vi "Process.vi"(8 "error in (no error)":errorcluster, 10 "Start State in":refnum<class "Start State.lvclass">, 11 "Architecture.lvlib:Thread.lvclass":refnum<class "Thread.lvclass">) -> (0 "error out":errorcluster, 1 "Stop?":bool, 3 "Architecture.lvlib:Thread.lvclass 2":refnum<class "Thread.lvclass">)   [LabVIEW 2019, in "Car Wash Controller.lvlib" / "Start State.lvclass"]
uses:
  Start State.lvclass
  Message/Message.lvclass
  Thread/Thread.lvclass
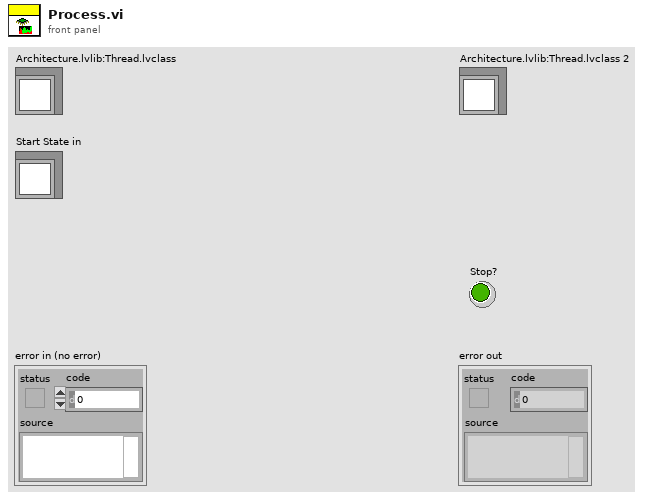
[diagram p1: front panel]
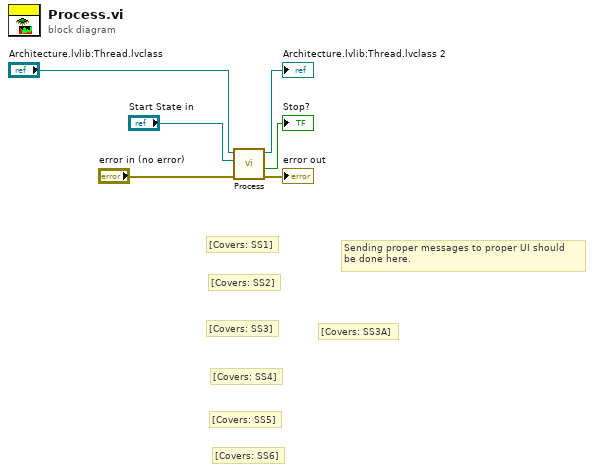
[diagram p0: block diagram]
diagram:
  # "[Covers: SS3A]"
  # "Sending proper messages to proper UI should\nbe done here."
  # "[Covers: SS6]"
  # "[Covers: SS5]"
  # "[Covers: SS4]"
  # "[Covers: SS3]"
  # "[Covers: SS2]"
  # "[Covers: SS1]"
  n1 = call-parent "Process.vi"("error in (no error)"="error in (no error)", "Message in"="Start State in", "Architecture.lvlib:Thread.lvclass"="Architecture.lvlib:Thread.lvclass") -> ("error out"=→"error out":errorcluster, "Stop?"=→"Stop?":bool, "Architecture.lvlib:Thread.lvclass 2"=→"Architecture.lvlib:Thread.lvclass 2":refnum<class "Thread.lvclass">)  [unwired: 6 in]
